vi "MouseMoveX.vi"(10 "Delta":i32, 11 "XYGraph输入":refnum<vi>) -> ()   [LabVIEW 2015]
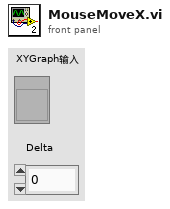
[diagram p1: front panel]
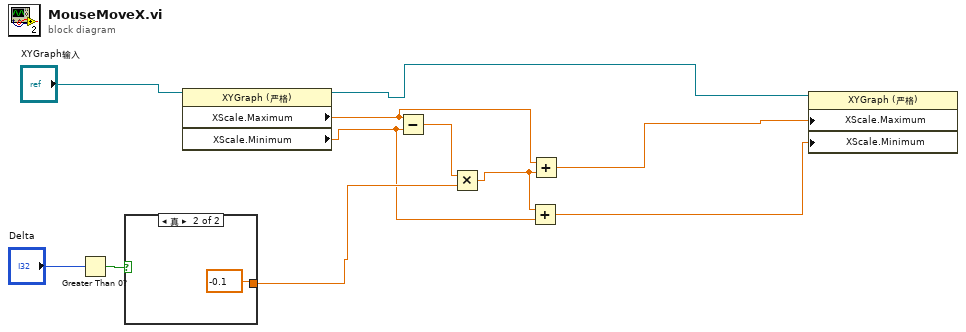
[diagram p0: block diagram]
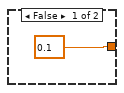
[diagram p2: hidden frame]
diagram:
  n1 = Greater Than 0?(x="Delta") -> (x > 0?=w11:bool)
  n2 = case shown="真" w11 {
    tunnel: [0.1 -0.1] -> w6
    frame False {
    }
    frame True {
    }
  }
  n3 = property class="XYGraph (严格)"(reference="XYGraph输入") -> (reference out=w8:refnum<vi>, "XScale.Maximum"=w5:dbl, "XScale.Minimum"=w2:dbl)  [unwired: 1 in, 1 out]
  n4 = Subtract(x=w5, y=w2) -> (x-y=w7:dbl)
  n5 = Multiply(x=w7, y=w6) -> (x*y=w3:dbl)
  n6 = Add(x=w3, y=w2) -> (x+y=w1:dbl)
  n7 = Add(x=w5, y=w3) -> (x+y=w4:dbl)
  n8 = property class="XYGraph (严格)"(reference=w8, "XScale.Maximum"=w4, "XScale.Minimum"=w1) -> ()  [unwired: 1 in, 2 out]
